vi "Menu parsing.vi"(9 "Menu Item":string, 10 "All devices":string[](array[string]), 11 "ItemPath":string) -> (2 "Item Path 2":string, 3 "ItemPath":string)   [LabVIEW 2020]
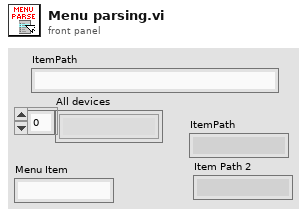
[diagram p1: front panel]
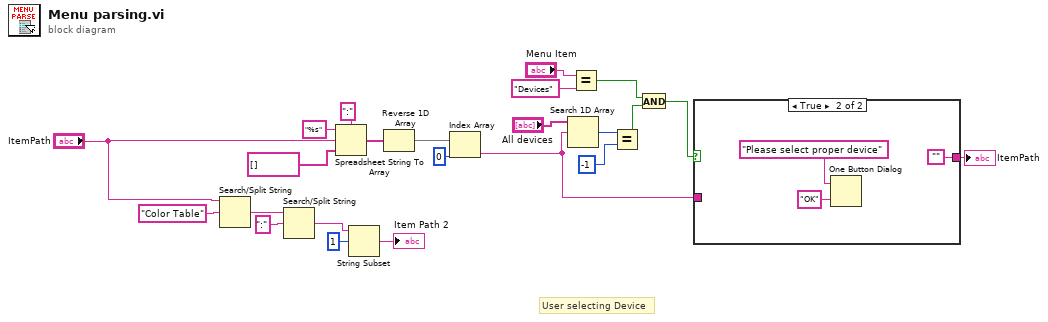
[diagram p0: block diagram]
diagram:
  # "User selecting Device"
  n1 = Search/Split String(string="ItemPath", search string/char (-)="Color Table") -> (match + rest of string=w13:string)  [unwired: 1 in, 2 out]
  n2 = Search/Split String(string=w13, search string/char (-)=":") -> (match + rest of string=w12:string)  [unwired: 1 in, 2 out]
  n3 = Spreadsheet String To Array(delimiter (Tab)=":", format string="%s", spreadsheet string="ItemPath", array type (2D Dbl)=string[] []) -> (array=w17:string[])
  n4 = String Subset(string=w12, offset (0)=1) -> (substring=→"Item Path 2":string)  [unwired: 1 in]
  n5 = Reverse 1D Array(array=w17) -> (reversed array=w16:string[])
  n6 = Index Array(array=w16, index=0) -> (element=w1:string)
  n7 = Search 1D Array(1D array="All devices", element=w1) -> (index of element=w7:i32)  [unwired: 1 in]
  n8 = Equal?(x="Menu Item", y="Devices") -> (x = y?=w4:bool)
  n9 = Equal?(x=w7, y=-1) -> (x = y?=w5:bool)
  n10 = And(x=w4, y=w5) -> (x .and. y?=w3:bool)
  n11 = case shown="True" w3 {
    tunnel: w1 -> [w24 _]
    tunnel: [w24 ""] -> w21
    frame False {
    }
    frame True {
      n12 = One Button Dialog(message="Please select proper device", button name ("OK")="OK") -> ()  [unwired: 1 out]
    }
  }
  "ItemPath" <- w21
